vi "CSDB_Config.mapping.vi"(1 "setMapping":bool, 2 "useMapping":bool, 3 "mapping":string[][](array[string]), 5 "error in (no error)":errorcluster) -> (16 "useMapping out":bool, 17 "mapping out":string[][](array[string]), 19 "error out":errorcluster)   [LabVIEW 2014, in "CSDB_Config.lvlib"]
doc: "Sets/Gets the mapping of an object."
uses:
  CSDB_Config.lvlib
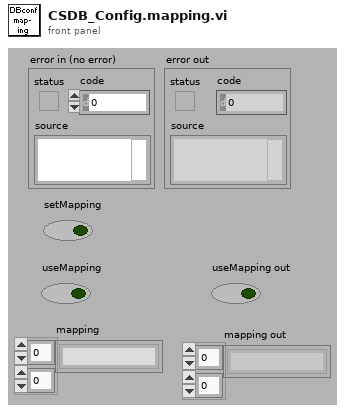
[diagram p1: front panel]
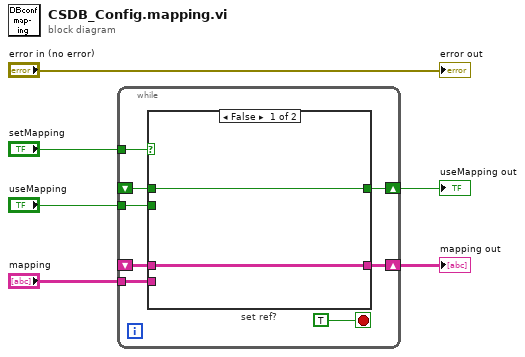
[diagram p0: block diagram]
diagram:
  n1 = while {
    tunnel: "setMapping" -> [w13]
    shift-right: [w11] -> w3
    shift-left: _ -> [w10]
    tunnel: "useMapping" -> [w12]
    shift-right: [w9] -> w1
    shift-left: _ -> [w7]
    tunnel: "mapping" -> [w8]
    stop <- TRUE stop-if-true
    n2 = case "set ref?" shown="False" w13 {
      tunnel: [w16 w18] -> w11
      tunnel: w12 -> [_ w18]
      tunnel: w10 -> [w16 _]
      tunnel: [w15 w17] -> w9
      tunnel: w8 -> [_ w17]
      tunnel: w7 -> [w15 _]
      frame False {
      }
      frame True {
      }
    }
  }
  "useMapping out" <- w3
  "mapping out" <- w1
  "error out" <- "error in (no error)"
